vi "Compile Digital Pattern Gen 1.3 Data.vi"(8 "error in (no error)":errorcluster, 11 "Device Item Ref in":T3 format="%.0x") -> (0 "error out":errorcluster, 1 "bitfile names":string[](array[string]), 2 "Digital Pattern Gens":T1[](array[typedef]), 3 "Device Item Ref out":T3 format="%.0x")   [LabVIEW 2013, in "Engine Simulation Toolkit System Explorer.lvlib"]
uses:
  Engine Simulation Toolkit System Explorer.lvlib
  <vilib>/NI Veristand/Custom Device API/Custom Device Item Ref.ctl
  Shared/1.3 Digital Pattern Gen Engine Data.ctl
  Shared/1.3 Digital Pattern Gen FIFO Idxs.ctl
  Digital Pattern Find Events Enum.ctl
  Shared/Constants and GUIDs.vi
  <vilib>/NI Veristand/Custom Device Tools/Custom Device Utility Library/NI VeriStand - Search for Item by GUID.vi
  <vilib>/NI Veristand/Custom Device Tools/Custom Device Utility Library/Custom Device Utility Library.lvlib
  Shared/Engine Simulation Toolkit Shared.lvlib
  <vilib>/NI Veristand/Custom Device API/Custom Device API.lvlib
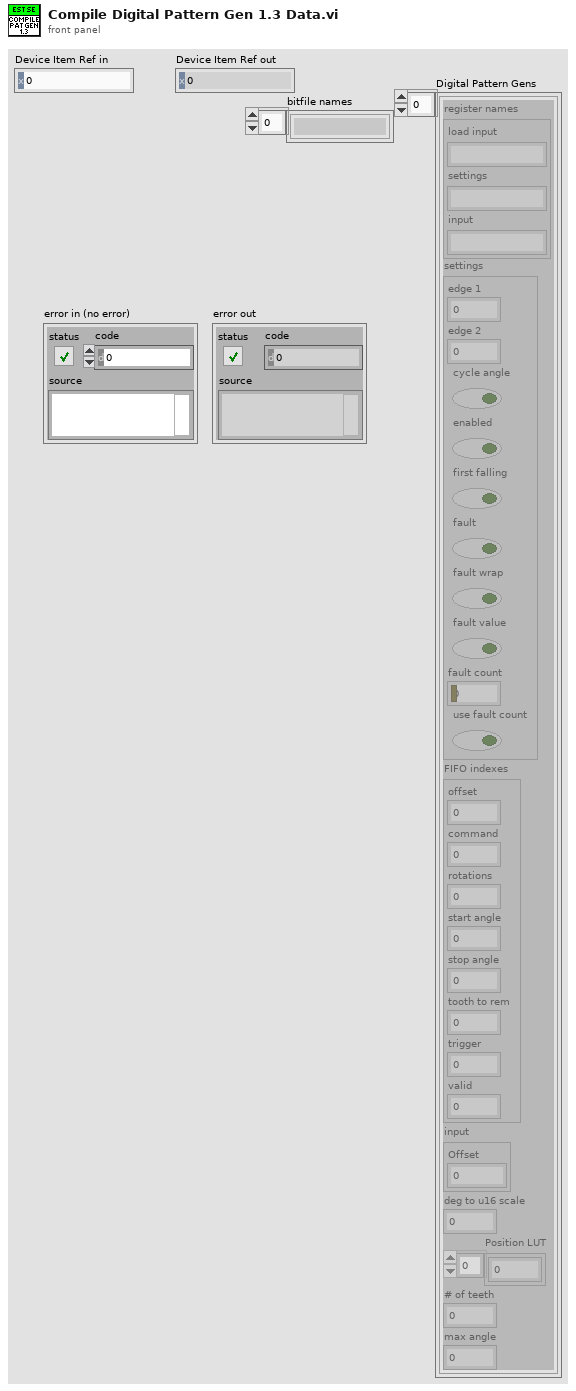
[diagram p1: front panel]
types:
  T1 = typedef "Engine Simulation Toolkit Shared.lvlib/1.3 Digital Pattern Gen Engine Data.ctl" = cluster{"register names":cluster{"load input":string, "settings":string, "input":string}, "settings":cluster{"edge 1":u16, "edge 2":u16, "cycle angle":bool, "enabled":bool, "first falling":bool, "fault":bool, "fault wrap":bool, "fault value":bool, "fault count":fxp<+,4,4>, "use fault count":bool}, "FIFO indexes":T2, "input":cluster{"Offset":i16}, "deg to u16 scale":dbl, "Position LUT":u16[], "# of teeth":i16, "max angle":dbl}
  T2 = typedef "Engine Simulation Toolkit Shared.lvlib/1.3 Digital Pattern Gen FIFO Idxs.ctl" = cluster{"offset":i32, "command":i32, "rotations":i32, "start angle":i32, "stop angle":i32, "tooth to rem":i32, "trigger":i32, "valid":i32}
  T3 = typedef "Custom Device API.lvlib/Custom Device Item Ref.ctl" = u64
  T4 = typedef "Engine Simulation Toolkit Shared.lvlib/Channel.ctl" = cluster{"Name":string, "Units":string, "Default":dbl, "Description":string}
  T5 = typedef "Engine Simulation Toolkit System Explorer.lvlib/Digital Pattern.ctl" = cluster{"Name":string, "Base":T6, "Remove":T7[], "Add":T8[], "FPGA Resource":string}
  T6 = typedef "Engine Simulation Toolkit System Explorer.lvlib/Digital Pattern Base.ctl" = cluster{"Length":dbl, "Teeth":u16, "Width":dbl, "Offset":dbl}
  T7 = typedef "Engine Simulation Toolkit System Explorer.lvlib/Digital Pattern Remove Edge.ctl" = cluster{"Tooth":u16, "Edge":bool}
  T8 = typedef "Engine Simulation Toolkit System Explorer.lvlib/Digital Pattern Add Pulse.ctl" = cluster{"Tooth":u16, "Offset":dbl, "Width":dbl}
  T9 = typedef "Engine Simulation Toolkit System Explorer.lvlib/Digital Pattern Find Events Enum.ctl" = enum16{"Rising Edge", "Falling Edge", "Any Edge", "Center Tooth", "Center Gap"}
  T10 = typedef "Engine Simulation Toolkit System Explorer.lvlib/Digital Pattern Expanded.ctl" = cluster{"X":dbl[], "Y":dbl[]}
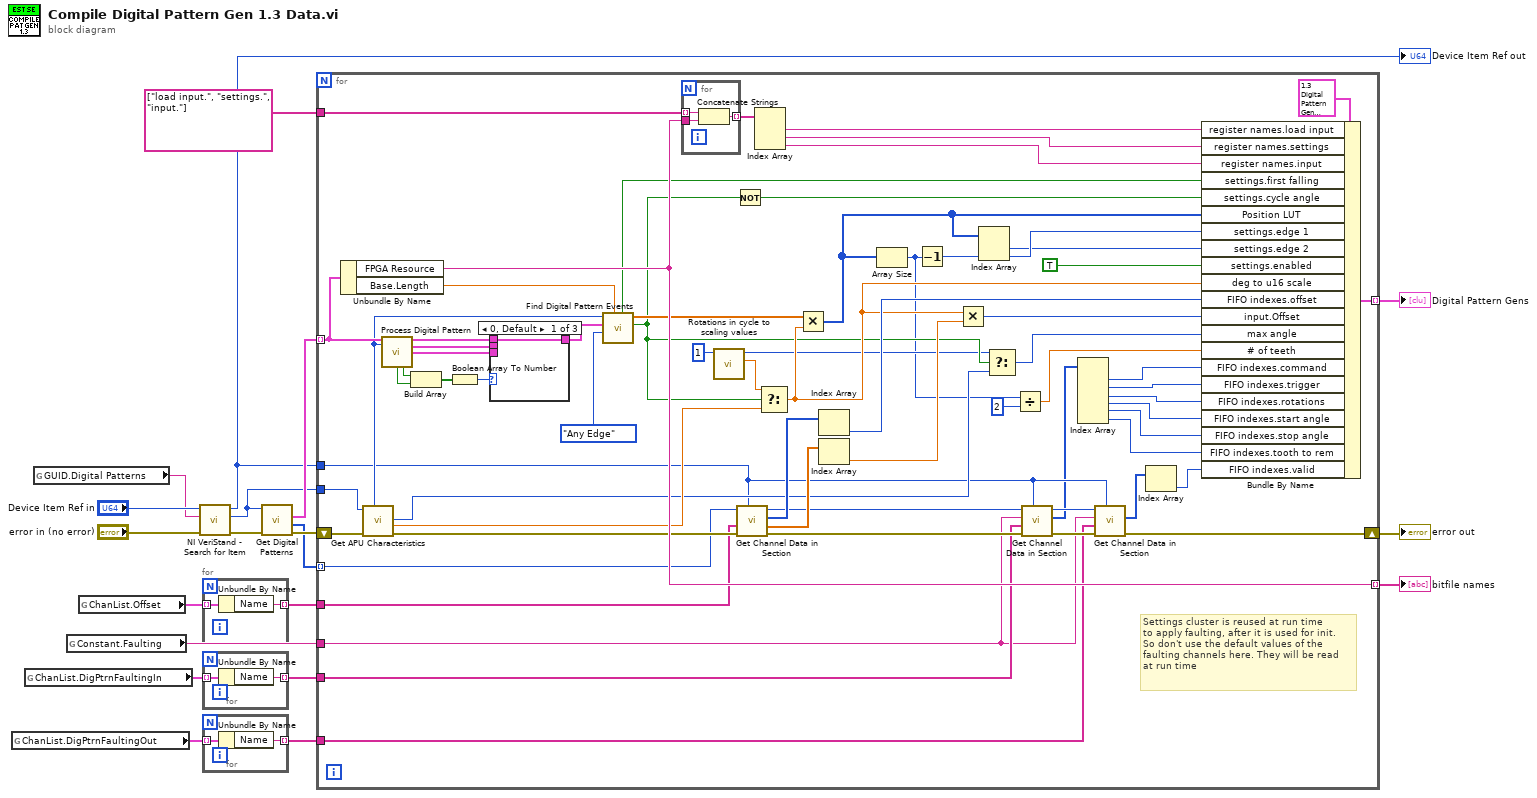
[diagram p0: block diagram]
diagram:
  n1 = global read "Constants and GUIDs.vi" "ChanList.DigPtrnFaultingOut"() -> (w4:T4[])
  n2 = global read "Constants and GUIDs.vi" "ChanList.DigPtrnFaultingIn"() -> (w5:T4[])
  n3 = global read "Constants and GUIDs.vi" "GUID.Digital Patterns"() -> (w18:string)
  n4 = global read "Constants and GUIDs.vi" "Constant.Faulting"() -> (w3:string)
  n5 = global read "Constants and GUIDs.vi" "ChanList.Offset"() -> (w7:T4[])
  n6 = call-poly <vilib>:"NI VeriStand - Search for Item.vi"("error in"="error in (no error)", "Item GUID"=w18, "Section Ref in"="Device Item Ref in") -> ("error out"=w17:errorcluster, "Item Ref"=w9:T3, "Section Ref out"=w10:T3)  [unwired: 5 in, 1 out]
  "Device Item Ref out" <- w10
  n7 = for {
    tunnel: [w22] -> w6 mode=indexing
    tunnel: w7 -> [w21] mode=indexing
    n8 = Unbundle By Name(w21) -> ("Name"=w22:string)
  }
  n9 = for {
    tunnel: [w24] -> w2 mode=indexing
    tunnel: w5 -> [w23] mode=indexing
    n10 = Unbundle By Name(w23) -> ("Name"=w24:string)
  }
  n11 = for {
    tunnel: [w26] -> w1 mode=indexing
    tunnel: w4 -> [w25] mode=indexing
    n12 = Unbundle By Name(w25) -> ("Name"=w26:string)
  }
  n13 = call "Get Digital Patterns.vi"("error in (no error)"=w17, "Item Ref in"=w9) -> ("error out"=w12:errorcluster, "references"=w8:T3[], "Patterns"=w11:T5[])  [unwired: 7 in]
  n14 = for {
    shift-right: [w27] -> w15
    shift-left: w12 -> [w84]
    tunnel: w11 -> [w82] mode=indexing
    tunnel: string[] ["load input.", "settings.", "input."] -> [w93]
    tunnel: [w88] -> w14 mode=indexing
    tunnel: [w86] -> w13 mode=indexing
    tunnel: w10 -> [w37]
    tunnel: w9 -> [w83]
    tunnel: w8 -> [w71] mode=indexing
    tunnel: w6 -> [w70]
    tunnel: w3 -> [w39]
    tunnel: w2 -> [w40]
    tunnel: w1 -> [w38]
    # "Settings cluster is reused at run time\nto apply faulting, after it is used for init.\nSo don't use the default values of the\nfaulting channels here. They will be read\nat run time"
    n15 = Unbundle By Name(w82) -> ("FPGA Resource"=w86:string, "Base.Length"=w80:dbl)
    n16 = call "Get APU Characteristics.vi"("error in (no error)"=w84, "Item Ref in"=w83) -> ("error out"=w78:errorcluster, "angle to u16 scale factor"=w54:dbl, "total angle span (degrees)"=w49:u16, "rotations"=w81:u16)  [unwired: 3 in, 3 out]
    n17 = call "Process Digital Pattern.vi"("EPT Pattern"=w82, "Rotations"=w81) -> ("Base"=w58:T10, 6:"Reduced"=w57:T10, 8:"Final"=w56:T10, 13:"Final"=w61:bool, 14:"Reduced"=w62:bool)  [unwired: 7 in, 2 out]
    n18 = Build Array(w62, w61) -> (w60:bool[])
    n19 = Boolean Array To Number(Boolean array=w60) -> (number=w59:u32)
    n20 = case shown="0, Default" w59 {
      tunnel: w58 -> [w94 _ _]
      tunnel: w57 -> [_ w95 _]
      tunnel: w56 -> [_ _ w96]
      tunnel: [w94 w95 w96] -> w55
      frame 0, Default {
      }
      frame 1 {
      }
      frame 2, 3 {
      }
    }
    n21 = call "Find Digital Pattern Events.vi"("Base.length"=w80, "Event"=Digital_Pattern_Find_Events_Enum."Any Edge", "Pattern"=w55, "Rotations"=w81) -> ("crank angle"=w51:bool, "Locations"=w77:dbl[], "first falling"=w52:bool)  [unwired: 5 in]
    n22 = for {
      tunnel: w86 -> [w99]
      tunnel: w93 -> [w98] mode=indexing
      tunnel: [w97] -> w91 mode=indexing
      n23 = Concatenate Strings(w98, w99) -> (w97:string)
    }
    n24 = call "Rotations in cycle to scaling values.vi"("rotations in a cycle"=u16 1) -> ("angle to u16 scale factor"=w53:dbl, "total angle span (degrees)"=w50:u16)  [unwired: 8 in, 1 out]
    n25 = Not(x=w51) -> (.not. x?=w63:bool)
    n26 = call "Get Channel Data in Section.vi"("Custom device ref"=w37, "error in (no error)"=w78, "Channels"=w70, "Item Ref in"=w71) -> ("error out"=w44:errorcluster, "default values"=w67:dbl[], "FIFO indexes"=w69:i32[], "Item Ref out"=w43:T3)  [unwired: 3 in, 1 out]
    n27 = Index Array(array=w91) -> (element #1=w90:string, element #2=w89:string, element #3=w87:string)  [unwired: 3 in]
    n28 = Select(t=w53, s=w51, f=w54) -> (s? t:f=w65:dbl)
    n29 = Multiply(x=w77, y=w65) -> (x*y=w72:u16[])
    n30 = Index Array(array=w69) -> (element=w68:i32)  [unwired: 1 in]
    n31 = Index Array(array=w67) -> (element=w66:dbl)  [unwired: 1 in]
    n32 = Array Size(array=w72) -> (size(s)=w47:i32)
    n33 = Decrement(x=w47) -> (x-1=w75:i32)
    n34 = Multiply(x=w65, y=w66) -> (x*y=w64:i16)
    n35 = Index Array(array=w72, index #2=w75) -> (element #1=w73:u16, element #2=w74:u16)  [unwired: 1 in]
    n36 = Select(t=w50, s=w51, f=w49) -> (s? t:f=w48:u16)
    n37 = Divide(x=w47, y=2) -> (x/y=w45:dbl)
    n38 = call "Get Channel Data in Section.vi"("Custom device ref"=w37, "error in (no error)"=w44, "Channels"=w40, "Section (\"\":none)"=w39, "Item Ref in"=w43) -> ("error out"=w42:errorcluster, "FIFO indexes"=w36:i32[], "Item Ref out"=w41:T3)  [unwired: 2 in, 2 out]
    n39 = Index Array(array=w36) -> (element #1=w35:i32, element #2=w34:i32, element #3=w33:i32, element #4=w32:i32, element #5=w31:i32, element #6=w30:i32)  [unwired: 6 in]
    n40 = call "Get Channel Data in Section.vi"("Custom device ref"=w37, "error in (no error)"=w42, "Channels"=w38, "Section (\"\":none)"=w39, "Item Ref in"=w41) -> ("error out"=w27:errorcluster, "FIFO indexes"=w29:i32[])  [unwired: 2 in, 3 out]
    n41 = Index Array(array=w29) -> (element=w28:i32)  [unwired: 1 in]
    n42 = Bundle By Name(cluster=T1 {"register names"={"load input"="", "settings"="", "input"=""}, "settings"={"edge 1"=0, "edge 2"=0, "cycle angle"=FALSE, "enabled"=FALSE, "first falling"=FALSE, "fault"=FALSE, "fault wrap"=FALSE, "fault value"=FALSE, "fault count"=0.0, "use fault count"=FALSE}, "FIFO indexes"={"offset"=0, "command"=0, "rotations"=0, "start angle"=0, "stop angle"=0, "tooth to rem"=0, "trigger"=0, "valid"=0}, "input"={"Offset"=0}, "deg to u16 scale"=0.0, "Position LUT"=[], "# of teeth"=0, "max angle"=0.0} ("1.0.0 Digital Pattern Gen"), "register names.load input"=w90, "register names.settings"=w89, "register names.input"=w87, "settings.first falling"=w52, "settings.cycle angle"=w63, "Position LUT"=w72, "settings.edge 1"=w74, "settings.edge 2"=w73, "settings.enabled"=TRUE, "deg to u16 scale"=w65, "FIFO indexes.offset"=w68, "input.Offset"=w64, "max angle"=w48, "# of teeth"=w45, "FIFO indexes.command"=w35, "FIFO indexes.trigger"=w34, "FIFO indexes.rotations"=w33, "FIFO indexes.start angle"=w32, "FIFO indexes.stop angle"=w31, "FIFO indexes.tooth to rem"=w30, "FIFO indexes.valid"=w28) -> (w88:T1)
  }
  "error out" <- w15
  "Digital Pattern Gens" <- w14
  "bitfile names" <- w13
